vi "PixelConvert.vi"(7 "lbPstPixelConvertParam":T1, 8 "pSrcData":u8[](array[numeric]), 9 "pDstBuf":u8[](array[numeric]), 10 "Interface handle":i64, 11 "error in (no error)":errorcluster) -> (1 "pDstBuf out":u8[](array[numeric]), 3 "error out":errorcluster)   [LabVIEW 2016]
uses:
  MVSDKmd.dll
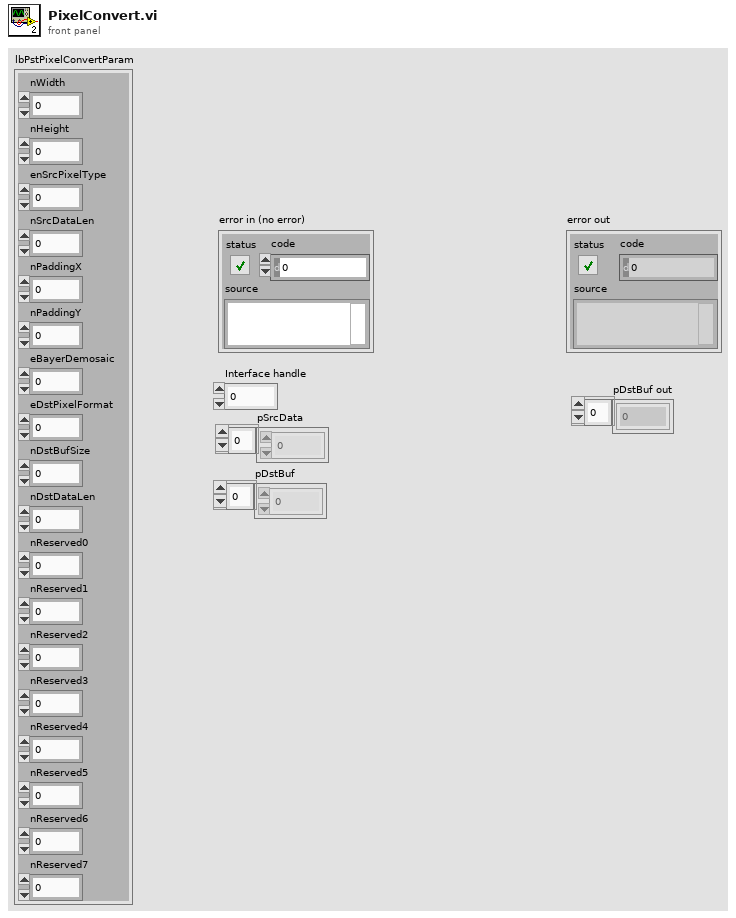
[diagram p1: front panel]
types:
  T1 = cluster{"nWidth":u32, "nHeight":u32, "enSrcPixelType":u32, "nSrcDataLen":u32, "nPaddingX":u32, "nPaddingY":u32, "eBayerDemosaic":u32, "eDstPixelFormat":u32, "nDstBufSize":u32, "nDstDataLen":u32, "nReserved0":u32, "nReserved1":u32, "nReserved2":u32, "nReserved3":u32, "nReserved4":u32, "nReserved5":u32, "nReserved6":u32, "nReserved7":u32}
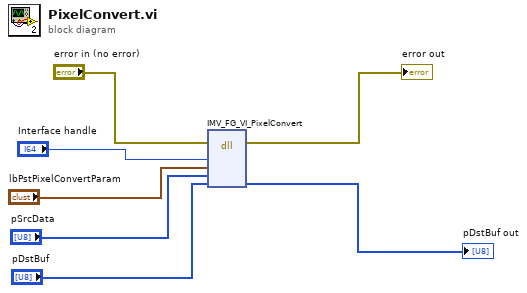
[diagram p0: block diagram]
diagram:
  n1 = dll-call lib="MVSDKmd.dll" fn="IMV_FG_VI_PixelConvert"(error in="error in (no error)", "interface handle"="Interface handle", "lbPstPixelConvertParam"="lbPstPixelConvertParam", "pSrcData"="pSrcData", "pDstBuf"="pDstBuf") -> (error out=→"error out":errorcluster, "pDstBuf"=→"pDstBuf out":u8[])  [unwired: 6 in, 1 out]
